vi "Measurement UI.vi"() -> ()   [LabVIEW 2021, in "audio_UI.lvlib"]
uses:
  audio_UI.lvlib
panel:
  in  "MeasGraphs":T1(tab)
  out "FreqDomainGraph":cluster{"x0":dbl, "dx":dbl, "magnitude":dbl[]}(graph) caption="AC"
  out "TimeDomainGraph":waveform(dbl)(graph) caption="AC"
  out "Channel":string
  out "Spectrum":dbl[](array[numeric])
  out "df":dbl
  out "f0":dbl
  out "Time domain":dbl[](array[numeric])
  out "dt":dbl
  out "THD+N":dbl
  out "THD":dbl
  out "SNR":dbl
  out "Calculated amplitude":dbl
  out "Calculated frequency":dbl
  out "SFDR":dbl
  out "Dynamic range":dbl
  out "Gain error":dbl
  in  "Analog source resource name":string
  in  "Protocol":string
  out "MeasTable":string[][](table)
  in  "OK Button":bool
  in  "Protocol":string(combo) caption="PROTOCOL"
  out "Calculated sample rate":u32 caption="SAMPLE RATE" format="%#.6pHz"
  in  "Protocol capture resource name":string caption="RESOURCE NAME"
  in  "Protocol settings":string="Protocol settings"
  in  "Analog source":string="Analog source "
  in  "Full scale range":dbl=3.16 caption="FULL SCALE RANGE" format="%.3pV"
  in  "Measurement settings":string="Measurement settings"
  in  "MeasSettingsOptions":i32(listbox)=-1
  in  "MeasSettings":bool
  in  "DSGResourceName":tag caption="RESOURCE NAME"
  in  "Weighting filter":T2(ring) caption="WEIGHTING FILTER"
  in  "Number of words":i32=19200 caption="NUMBER OF WORDS"
  in  "Clock rate":u32=12288000 caption="CLOCK RATE" format="%#.6pHz"
  in  "Band stop":dbl=20000.0 caption="BAND STOP" format="%#_6pHz"
  in  "Band start":dbl=20.0 caption="BAND START" format="%#_6pHz"
  in  "Amplitude":dbl=-1.0 caption="AMPLITUDE" format="%#_6pdB"
  in  "Frequency":dbl=1000.0 caption="FREQUENCY" format="%#_6pHz"
  in  "Sensitivity":dbl=0.34762 caption="SENSITIVITY" format="%.5fFS/Pa"
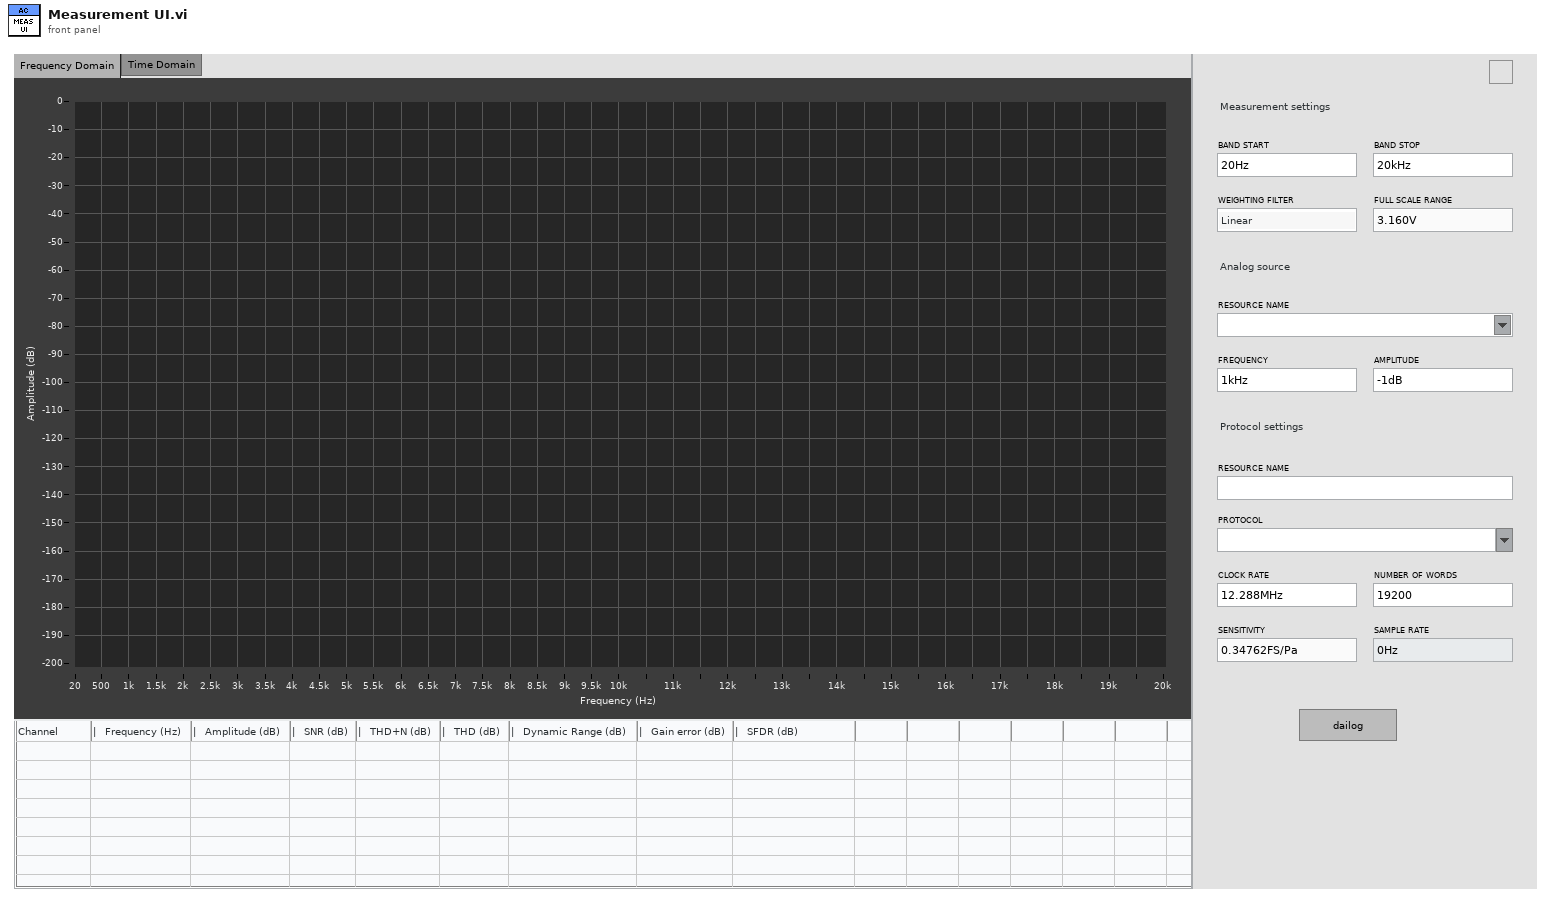
[diagram p1: front panel]
types:
  T1 = enum32{"Frequency Domain", "Time Domain", "Hidden Controls"}
  T2 = enum16{"Linear", "A-Weighting", "B-Weighting", "C-Weighting"}
  T3 = enum16{"open", "replace", "create", "open or create", "replace or create", "replace or create with confirmation"}
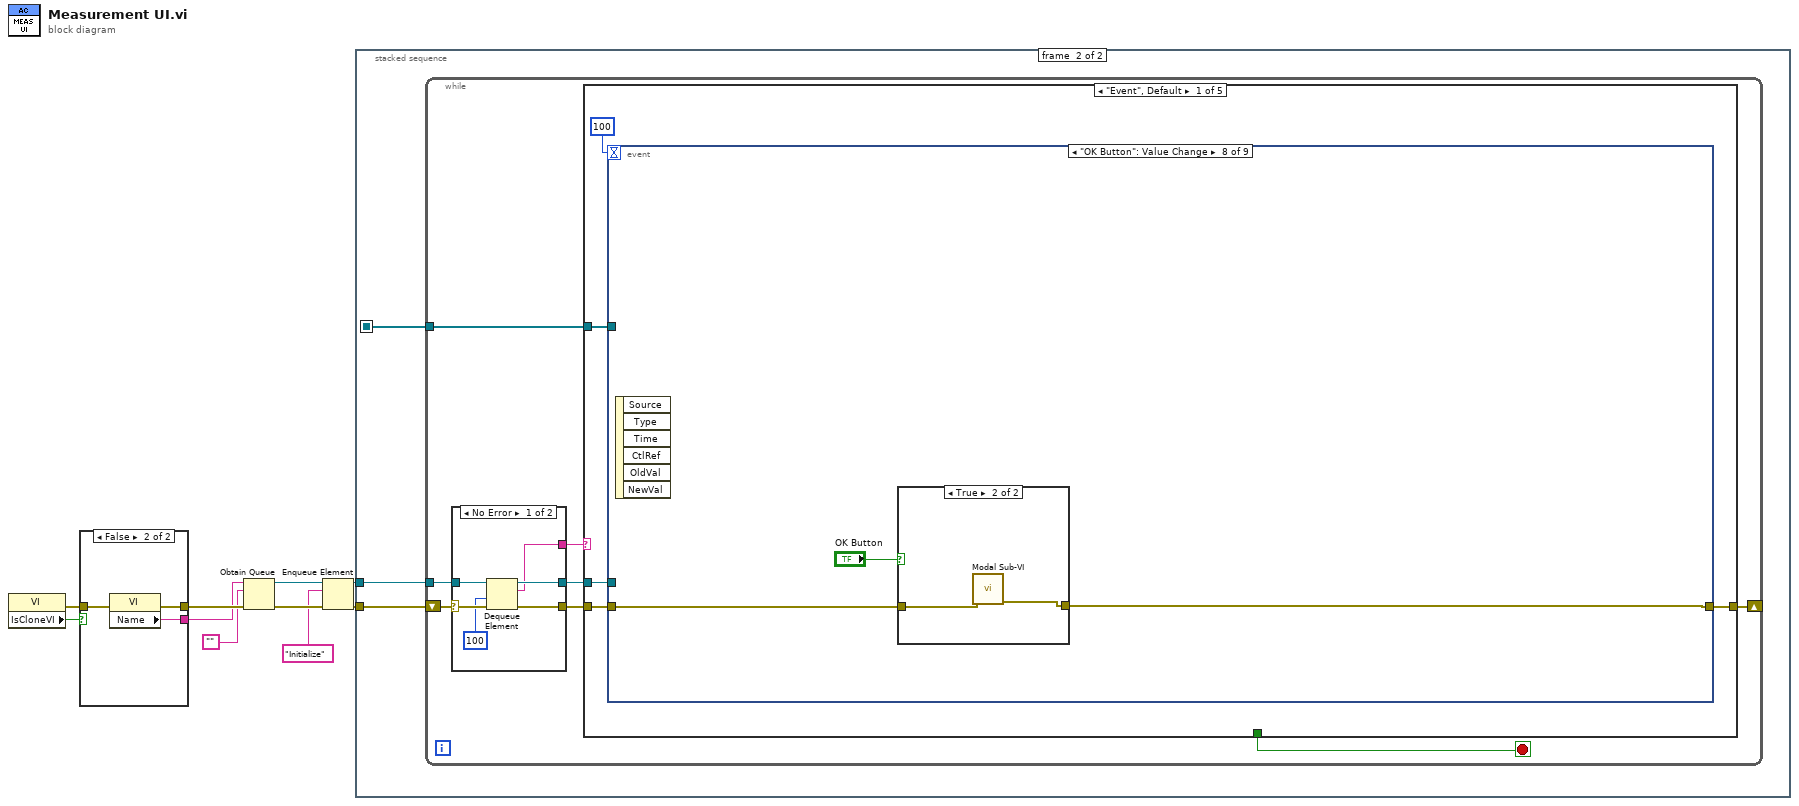
[diagram p0: block diagram]
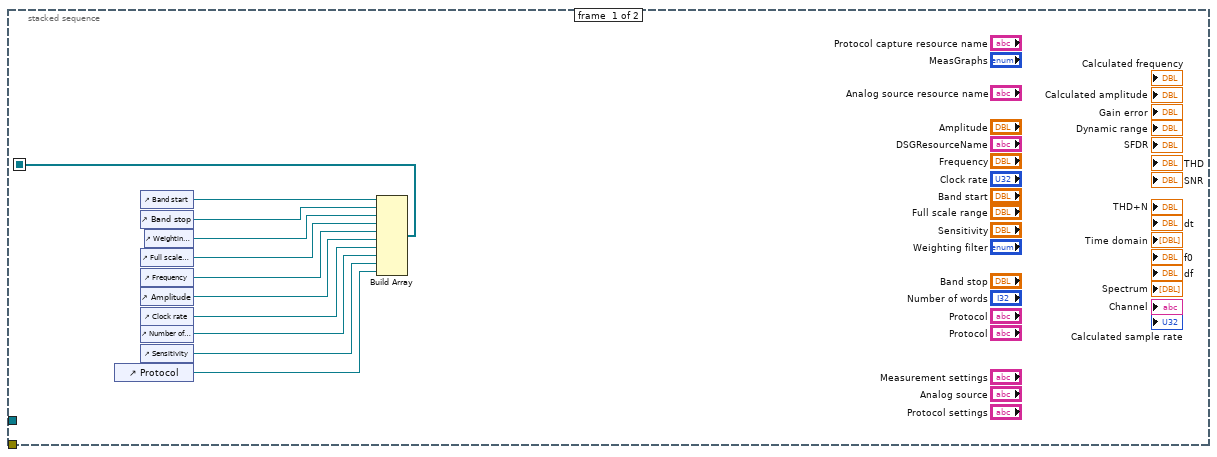
[diagram p2: hidden frame]
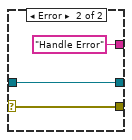
[diagram p3: hidden frame]
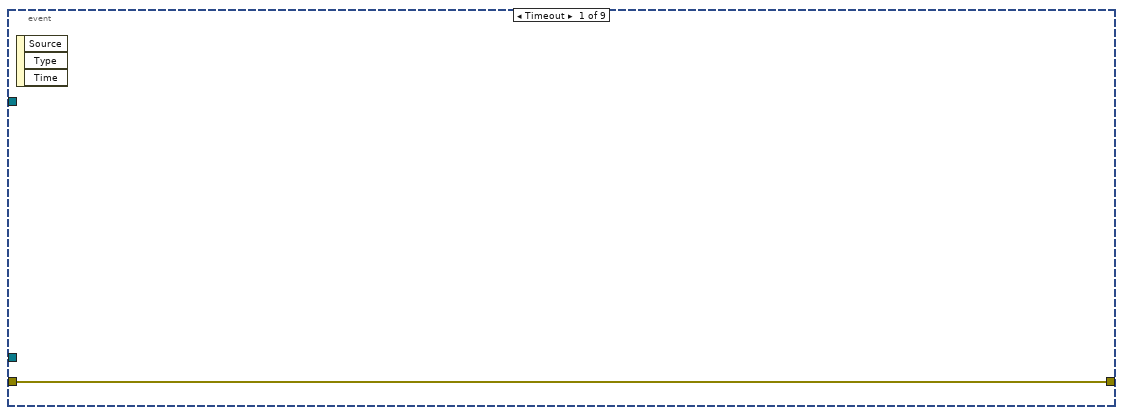
[diagram p4: hidden frame]
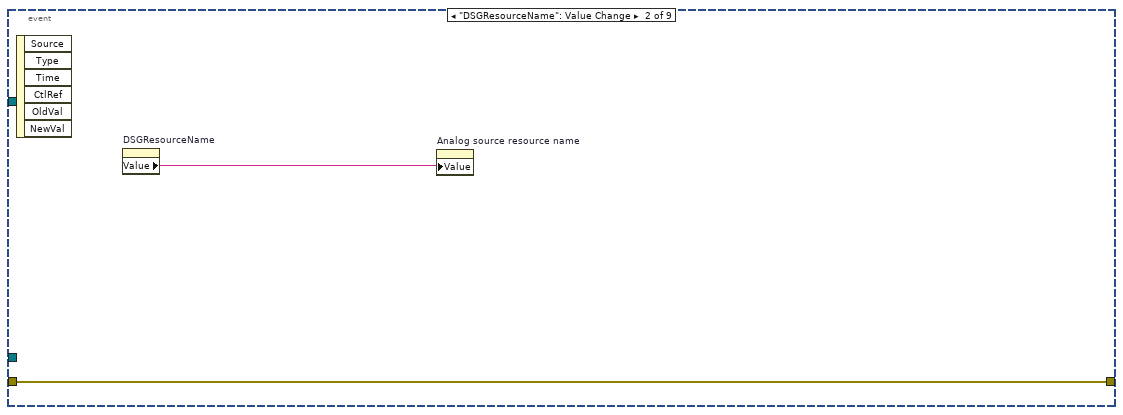
[diagram p5: hidden frame]
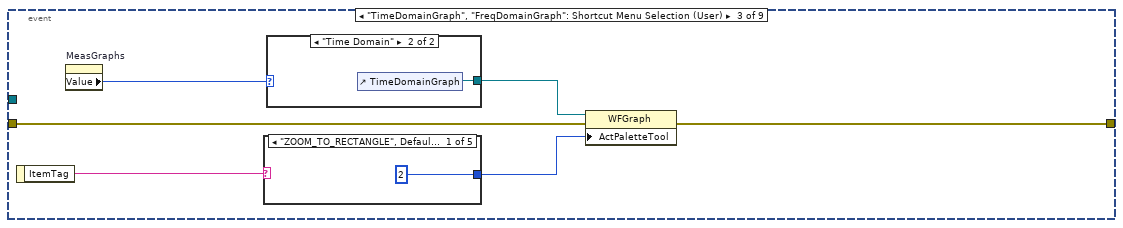
[diagram p6: hidden frame]
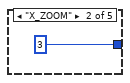
[diagram p7: hidden frame]
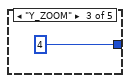
[diagram p8: hidden frame]
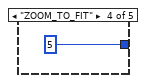
[diagram p9: hidden frame]
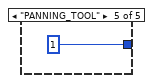
[diagram p10: hidden frame]
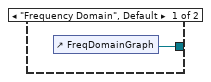
[diagram p11: hidden frame]
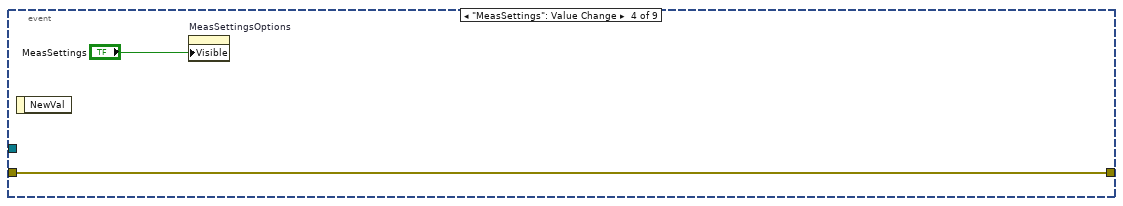
[diagram p12: hidden frame]
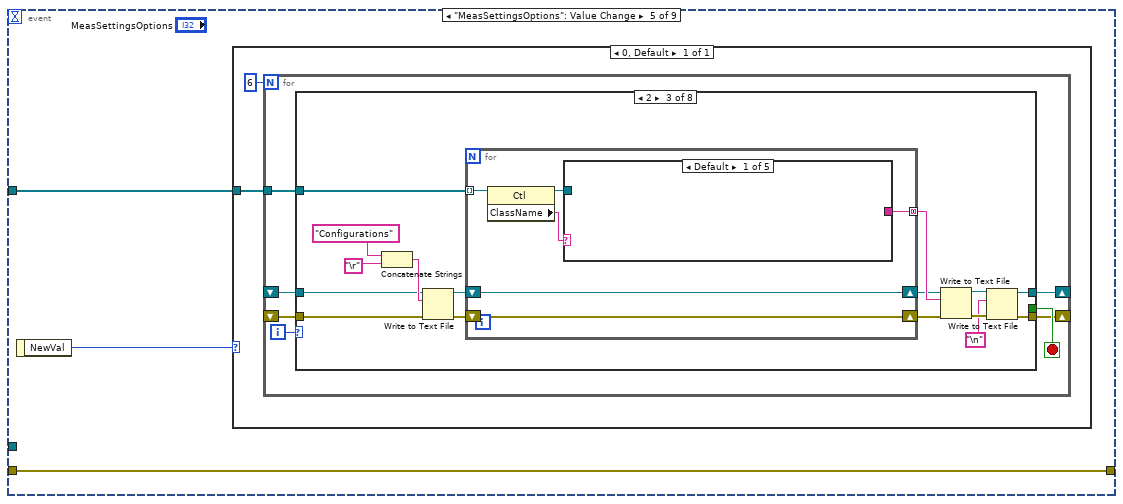
[diagram p13: hidden frame]
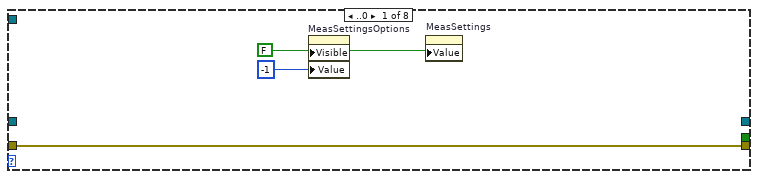
[diagram p14: hidden frame]
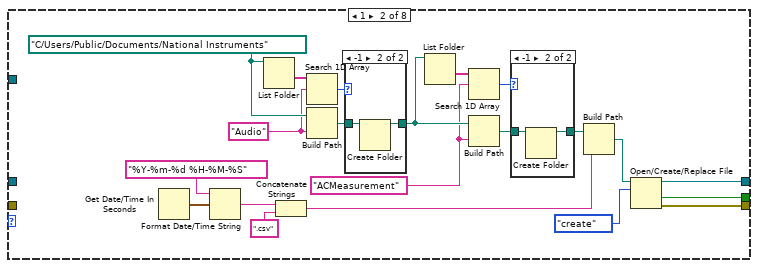
[diagram p15: hidden frame]
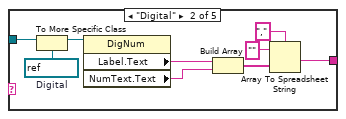
[diagram p18: hidden frame]
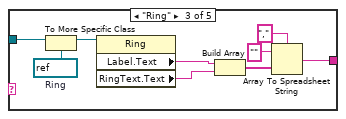
[diagram p19: hidden frame]
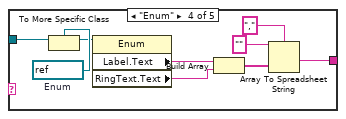
[diagram p20: hidden frame]
diagram:
  n1 = property on="Property Node" class="VI"() -> (error out=w1:errorcluster, "IsCloneVI"=w2:bool)  [unwired: 2 in, 1 out]
  n2 = case shown="False" w2 {
    tunnel: [w13 w16] -> w10
    tunnel: [w12 w15] -> w9
    tunnel: w1 -> [w11 w14]
    frame True {
      n3 = property on="Property Node" class="VI"(error in=w11) -> (error out=w13:errorcluster, "Clone Name"=w12:string)  [unwired: 1 in, 1 out]
    }
    frame False {
      n4 = property on="Property Node" class="VI"(error in=w14) -> (error out=w16:errorcluster, "Name"=w15:string)  [unwired: 1 in, 1 out]
    }
  }
  n5 = Obtain Queue(name (unnamed)=w9, element data type="" ("Empty String Constant"), error in (no error)=w10) -> (queue out=w6:refnum<queue>, error out=w8:errorcluster)  [unwired: 2 in, 1 out]
  n6 = Enqueue Element(queue=w6, element="Initialize", error in (no error)=w8) -> (queue out=w5:refnum<queue>, error out=w7:errorcluster)  [unwired: 1 in, 1 out]
  n7 = stacked-sequence {
    seq-local: [w24 _] -> [_ w28]
    tunnel: w7 -> [_ w30]
    tunnel: w5 -> [_ w29]
    frame #0 {
      n8 = control-ref of="Protocol"() -> (w17:refnum<vi>)
      n9 = control-ref of="Band start"() -> (w27:refnum<vi>)
      n10 = control-ref of="Band stop"() -> (w26:refnum<vi>)
      n11 = control-ref of="Full scale range"() -> (w23:refnum<vi>)
      n12 = control-ref of="Frequency"() -> (w22:refnum<vi>)
      n13 = control-ref of="Amplitude"() -> (w21:refnum<vi>)
      n14 = control-ref of="Clock rate"() -> (w20:refnum<vi>)
      n15 = control-ref of="Number of words"() -> (w18:refnum<vi>)
      n16 = control-ref of="Sensitivity"() -> (w19:refnum<vi>)
      n17 = control-ref of="Weighting filter"() -> (w25:refnum<vi>)
      n18 = Build Array(w27, w26, w25, w23, w22, w21, w20, w18, w19, w17) -> (w24:refnum<vi>[])
    }
    frame #1 {
      n19 = while {
        shift-right: [w33] -> _
        shift-left: w30 -> [w38]
        tunnel: w29 -> [w36]
        tunnel: w28 -> [w31]
        stop <- w32 stop-if-true
        n20 = case shown="No Error" w38 {
          selector: w38 -> [w44 w47]
          tunnel: [w43 w47] -> w37
          tunnel: w36 -> [w42 w46]
          tunnel: [w41 w46] -> w35
          tunnel: [w40 "Handle Error"] -> w34
          frame No Error {
            n21 = Dequeue Element(queue=w42, timeout in ms (-1)=100, error in (no error)=w44) -> (queue out=w41:refnum<queue>, element=w40:string, error out=w43:errorcluster)  [unwired: 1 out]
          }
          frame Error {
          }
        }
        n22 = case shown="\"Event\", Default" w34 {
          tunnel: w37 -> [w51 w325 w366 w381 w382]
          tunnel: w35 -> [w49 _ _ w379 _]
          tunnel: [w52 w325 w366 w376 w382] -> w33
          tunnel: [_ _ _ TRUE _] -> w32
          tunnel: w31 -> [w48 _ _ _ _]
          frame "Event", Default {
            n23 = event shown="[7] \"OK Button\": Value Change" {
              selector: _ -> [_ _ _ _ _ _ _ _ _]
              dyn-events: _ -> [_ _ _ _ _ _ _ _ _]
              timeout: 100 -> [_ _ _ _ _ _ _ _ _]
              tunnel: [w53 w54 w58 _ w73 w275 w279 w300 w307] -> w52
              tunnel: w51 -> [w53 w54 w57 w69 w73 w275 w278 w301 w308]
              tunnel: w49 -> [_ _ _ _ _ _ _ _ w306]
              tunnel: [_ _ _ w69 _ _ _ _ _] -> _
              tunnel: w48 -> [_ _ _ _ w71 _ _ _ _]
              event Timeout {
                n24 = event-data() -> ()  [unwired: 1 in, 3 out]
              }
              event "DSGResourceName": Value Change {
                n25 = event-data() -> ()  [unwired: 1 in, 6 out]
                n26 = property on="DSGResourceName" class="DAQmxName"() -> ("Value"=w55:string)  [unwired: 2 in, 2 out]
                n27 = property on="Analog source resource name" class="Str"("Value"=w55) -> ()  [unwired: 2 in, 2 out]
              }
              event "TimeDomainGraph", "FreqDomainGraph": Shortcut Menu Selection (User) {
                n28 = event-data() -> ("ItemTag"=w60:string)  [unwired: 1 in]
                n29 = property on="MeasGraphs" class="TabCtl (strict)"() -> ("Value"=w61:T1)  [unwired: 2 in, 2 out]
                n30 = case shown="\"ZOOM_TO_RECTANGLE\", Default" w60 {
                  tunnel: [2 3 4 5 1] -> w56
                  frame "ZOOM_TO_RECTANGLE", Default {
                  }
                  frame "X_ZOOM" {
                  }
                  frame "Y_ZOOM" {
                  }
                  frame "ZOOM_TO_FIT" {
                  }
                  frame "PANNING_TOOL" {
                  }
                }
                n31 = case shown="\"Time Domain\"" w61 {
                  tunnel: [w67 w68] -> w59
                  frame "Frequency Domain", Default {
                    n32 = control-ref of="FreqDomainGraph"() -> (w67:refnum<vi>)
                  }
                  frame "Time Domain" {
                    n33 = control-ref of="TimeDomainGraph"() -> (w68:refnum<vi>)
                  }
                }
                n34 = property on="Property Node" class="WFGraph"(reference=w59, error in=w57, "ActPaletteTool"=w56) -> (error out=w58:errorcluster)  [unwired: 1 out]
              }
              event "MeasSettings": Value Change {
                n35 = event-data() -> ()  [unwired: 1 in, 1 out]
                n36 = property on="MeasSettingsOptions" class="LstBox (strict)"("Visible"="MeasSettings") -> ()  [unwired: 2 in, 2 out]
              }
              event "MeasSettingsOptions": Value Change {
                n37 = event-data() -> ("NewVal"=w72:i32)  [unwired: 1 in]
                n38 = case shown="0, Default" w72 {
                  tunnel: w71 -> [w74]
                  frame 0, Default {
                    n39 = for {
                      N: 6 -> [_]
                      shift-right: [w80] -> _
                      shift-left: _ -> [w79]
                      shift-right: [w78] -> _
                      shift-left: _ -> [w77]
                      tunnel: w74 -> [w76]
                      i -> [w82]
                      stop <- w81 stop-if-true
                      n40 = case shown="2" w82 {
                        tunnel: [_ w99 _ _ _ _ _ _] -> w81
                        tunnel: [_ w105 w125 w178 w205 w246 refnum<file> refnum ("refnum out") w274] -> w80
                        tunnel: w79 -> [_ _ w122 w189 w228 w247 w272 w274]
                        tunnel: [w83 w98 w124 w177 w203 w245 w270 w273] -> w78
                        tunnel: w77 -> [w83 _ w120 w188 w227 w248 w269 w273]
                        tunnel: w76 -> [_ _ w123 _ _ _ _ _]
                        frame ..0 {
                          w85 = FALSE ("Visible")
                          n41 = property on="MeasSettingsOptions" class="LstBox (strict)"("Visible"=w85, "Value"=-1 ("MeasSettingsOptions")) -> ()  [unwired: 2 in, 2 out]
                          n42 = property on="MeasSettings" class="Bool (strict)"("Value"=w85) -> ()  [unwired: 2 in, 2 out]
                        }
                        frame 1 {
                          w94 = "ACMeasurement" ("prompt")
                          w101 = "Audio" ("prompt")
                          w104 = path "C:/Users/Public/Documents/National Instruments" ("base path")
                          n43 = Get Date/Time In Seconds() -> (seconds since 1Jan1904=w91:timestamp)
                          n44 = Format Date/Time String(time format string (%c)="%Y-%m-%d %H-%M-%S", seconds (now)=w91) -> (date/time string=w90:string)  [unwired: 1 in]
                          n45 = List Folder(path=w104) -> (folder names=w102:string[])  [unwired: 3 in, 3 out]
                          n46 = Concatenate Strings(w90, ".csv" ("string")) -> (w87:string)
                          n47 = Search 1D Array(1D array=w102, element=w101) -> (index of element=w100:i32)  [unwired: 1 in]
                          n48 = Build Path(base path=w104, name or relative path=w101) -> (appended path=w103:path)
                          n49 = case shown="-1" w100 {
                            tunnel: w103 -> [w110 w112]
                            tunnel: [w110 w111] -> w95
                            frame Default {
                            }
                            frame -1 {
                              n50 = Create Folder(path (use dialog)=w112) -> (created path=w111:path)  [unwired: 2 in, 2 out]
                            }
                          }
                          n51 = List Folder(path=w95) -> (folder names=w97:string[])  [unwired: 3 in, 3 out]
                          n52 = Search 1D Array(1D array=w97, element=w94) -> (index of element=w96:i32)  [unwired: 1 in]
                          n53 = Build Path(base path=w95, name or relative path=w94) -> (appended path=w93:path)
                          n54 = case shown="-1" w96 {
                            tunnel: w93 -> [w107 w109]
                            tunnel: [w107 w108] -> w88
                            frame Default {
                            }
                            frame -1 {
                              n55 = Create Folder(path (use dialog)=w109) -> (created path=w108:path)  [unwired: 2 in, 2 out]
                            }
                          }
                          n56 = Build Path(base path=w88, name or relative path=w87) -> (appended path=w86:path)
                          n57 = Open/Create/Replace File(file path (use dialog)=w86, operation (0:open)=T3."create") -> (refnum out=w105:refnum<file>, cancelled=w99:bool, error out=w98:errorcluster)  [unwired: 4 in]
                        }
                        frame 2 {
                          n58 = Concatenate Strings("Configurations" ("format string"), "\r" ("Carriage Return Constant")) -> (w126:string)
                          n59 = Write to Text File(file (use dialog)=w122, text=w126, error in=w120) -> (refnum out=w119:refnum<file>, error out=w121:errorcluster)  [unwired: 1 in, 1 out]
                          n60 = for {
                            tunnel: w123 -> [w130] mode=indexing
                            shift-right: [w134] -> w117
                            shift-left: w119 -> [w134]
                            shift-right: [w133] -> w116
                            shift-left: w121 -> [w133]
                            tunnel: [w132] -> w118 mode=concatenating
                            n61 = property on="Property Node" class="Ctl"(reference=w130) -> (reference out=w131:refnum<vi>, "ClassName"=w129:string)  [unwired: 1 in, 1 out]
                            n62 = case shown="Default" w129 {
                              tunnel: [_ w138 w148 w157 w162] -> w132
                              tunnel: w131 -> [_ w136 w146 w161 w170]
                              frame Default {
                              }
                              frame "Digital" {
                                w135 = refnum<vi> refnum  # Digital
                                n63 = To More Specific Class(target class=w135, reference=w136) -> (specific class reference=w137:refnum<vi>)  [unwired: 1 in, 1 out]
                                n64 = property on="Property Node" class="DigNum"(reference=w137) -> ("Label.Text"=w143:string, "NumText.Text"=w142:string)  [unwired: 1 in, 2 out]
                                n65 = Build Array(w143, w142) -> (w139:string[])
                                n66 = Array To Spreadsheet String(delimiter (Tab)=",", array=w139, 3:"" ("format string")) -> (spreadsheet string=w138:string)
                              }
                              frame "Ring" {
                                w145 = refnum<vi> refnum  # Ring
                                n67 = To More Specific Class(target class=w145, reference=w146) -> (specific class reference=w147:refnum<vi>)  [unwired: 1 in, 1 out]
                                n68 = property on="Property Node" class="Ring"(reference=w147) -> ("Label.Text"=w144:string, "RingText.Text"=w152:string)  [unwired: 1 in, 2 out]
                                n69 = Build Array(w144, w152) -> (w149:string[])
                                n70 = Array To Spreadsheet String(delimiter (Tab)=",", array=w149, 3:"" ("format string")) -> (spreadsheet string=w148:string)
                              }
                              frame "Enum" {
                                w160 = refnum<vi> refnum  # Enum
                                n71 = To More Specific Class(target class=w160, reference=w161) -> (specific class reference=w156:refnum<vi>)  [unwired: 1 in, 1 out]
                                n72 = property on="Property Node" class="Enum"(reference=w156) -> ("Label.Text"=w155:string, "RingText.Text"=w154:string)  [unwired: 1 in, 2 out]
                                n73 = Build Array(w155, w154) -> (w153:string[])
                                n74 = Array To Spreadsheet String(delimiter (Tab)=",", array=w153, 3:"" ("format string")) -> (spreadsheet string=w157:string)
                              }
                              frame "ComboBox" {
                                w169 = refnum<vi> refnum  # ComboBox
                                n75 = To More Specific Class(target class=w169, reference=w170) -> (specific class reference=w168:refnum<vi>)  [unwired: 1 in, 1 out]
                                n76 = property class="CmbBox"(reference=w168) -> ("Label.Text"=w164:string, "Value"=w163:string)  [unwired: 1 in, 2 out]
                                n77 = Build Array(w164, w163) -> (w167:string[])
                                n78 = Array To Spreadsheet String(delimiter (Tab)=",", array=w167, 3:"" ("format string")) -> (spreadsheet string=w162:string)
                              }
                            }
                          }
                          n79 = Write to Text File(file (use dialog)=w117, text=w118, error in=w116) -> (refnum out=w115:refnum<file>, error out=w114:errorcluster)  [unwired: 1 in, 1 out]
                          n80 = Write to Text File(file (use dialog)=w115, text="\n" ("Line Feed Constant"), error in=w114) -> (refnum out=w125:refnum<file>, error out=w124:errorcluster)  [unwired: 1 in, 1 out]
                        }
                        frame 3 {
                          n81 = property on="MeasTable" class="Tbl (strict)"() -> ("Column Headers[]"=w172:string[], "Value"=w171:string[][])  [unwired: 2 in, 2 out]
                          n82 = Build Array (concatenate)(w172, w171) -> (w186:string[][])
                          n83 = for {
                            tunnel: w186 -> [w191] mode=indexing
                            tunnel: [w190] -> w185 mode=indexing
                            n84 = for {
                              tunnel: w191 -> [w193] mode=indexing
                              tunnel: [w192] -> w190 mode=indexing
                              n85 = Match Pattern(string=w193, regular expression="|") -> (before substring=w197:string, after substring=w196:string, offset past match=w199:i32)  [unwired: 1 in, 1 out]
                              n86 = Less Than 0?(x=w199) -> (x < 0?=w198:bool)
                              n87 = Select(t=w197, s=w198, f=w196) -> (s? t:f=w195:string)
                              n88 = Match Pattern(string=w195, regular expression="[\\t\\n\\r\\s]*$") -> (before substring=w192:string)  [unwired: 1 in, 3 out]
                            }
                          }
                          n89 = Concatenate Strings("Results" ("element"), "\r" ("Carriage Return Constant")) -> (w173:string)
                          n90 = Write to Text File(file (use dialog)=w189, text=w173, error in=w188) -> (refnum out=w187:refnum<file>, error out=w181:errorcluster)  [unwired: 1 in, 1 out]
                          n91 = Array To Spreadsheet String(delimiter (Tab)=",", array=w185, 3:"" ("format string")) -> (spreadsheet string=w182:string)
                          n92 = Write to Text File(file (use dialog)=w187, text=w182, error in=w181) -> (refnum out=w180:refnum<file>, error out=w179:errorcluster)  [unwired: 1 in, 1 out]
                          n93 = Write to Text File(file (use dialog)=w180, text="\n" ("Line Feed Constant"), error in=w179) -> (refnum out=w178:refnum<file>, error out=w177:errorcluster)  [unwired: 1 in, 1 out]
                        }
                        frame 4 {
                          n94 = property on="FreqDomainGraph" class="WFGraph (strict)"() -> ("Value"=w208:cluster{"x0":dbl, "dx":dbl, "magnitude":dbl[]})  [unwired: 2 in, 2 out]
                          n95 = Concatenate Strings("Frequency Domain" ("string"), "\r" ("Carriage Return Constant")) -> (w225:string)
                          n96 = Build Array("Frequency (Hz)", "Amplitude (dB)") -> (w224:string[])
                          n97 = Write to Text File(file (use dialog)=w228, text=w225, error in=w227) -> (refnum out=w221:refnum<file>, error out=w220:errorcluster)  [unwired: 1 in, 1 out]
                          n98 = Unbundle By Name(w208) -> ("dx"=w212:dbl, "x0"=w213:dbl, "magnitude"=w211:dbl[])
                          n99 = Array To Spreadsheet String(delimiter (Tab)=",", array=w224, 3:"" ("format string")) -> (spreadsheet string=w219:string)
                          n100 = Write to Text File(file (use dialog)=w221, text=w219, error in=w220) -> (refnum out=w218:refnum<file>, error out=w217:errorcluster)  [unwired: 1 in, 1 out]
                          n101 = for {
                            tunnel: w211 -> [w232] mode=indexing
                            tunnel: w212 -> [w236]
                            tunnel: w213 -> [w234]
                            tunnel: [w229] -> w214 mode=indexing
                            i -> [w237]
                            n102 = Multiply(x=w237, y=w236) -> (x*y=w235:dbl)
                            n103 = Add(x=w235, y=w234) -> (x+y=w233:dbl)
                            n104 = Format Into String(w233) -> (resulting string=w230:string)  [unwired: 3 in, 1 out]
                            n105 = Format Into String(w232) -> (resulting string=w231:string)  [unwired: 3 in, 1 out]
                            n106 = Build Array(w230, w231) -> (w229:string[])
                          }
                          n107 = Array To Spreadsheet String(delimiter (Tab)=",", array=w214, 3:"" ("format string")) -> (spreadsheet string=w210:string)
                          n108 = Write to Text File(file (use dialog)=w218, text=w210, error in=w217) -> (refnum out=w207:refnum<file>, error out=w206:errorcluster)  [unwired: 1 in, 1 out]
                          n109 = Write to Text File(file (use dialog)=w207, text="\n" ("Line Feed Constant"), error in=w206) -> (refnum out=w205:refnum<file>, error out=w203:errorcluster)  [unwired: 1 in, 1 out]
                        }
                        frame 5 {
                          n110 = property on="TimeDomainGraph" class="WFGraph (strict)"() -> ("Value"=w244:waveform(dbl))  [unwired: 2 in, 2 out]
                          n111 = Concatenate Strings("Time Domain" ("string"), "\r" ("Carriage Return Constant")) -> (w260:string)
                          n112 = Write to Text File(file (use dialog)=w247, text=w260, error in=w248) -> (refnum out=w257:refnum<file>, error out=w256:errorcluster)  [unwired: 1 in, 1 out]
                          n113 = Build Array("Time (s)", "Amplitude (V)") -> (w259:string[])
                          n114 = Unbundle By Name ("Get Waveform Components")(w244) -> ("dt"=w242:dbl, "Y"=w243:dbl[])
                          n115 = Array To Spreadsheet String(delimiter (Tab)=",", array=w259, 3:"" ("format string")) -> (spreadsheet string=w255:string)
                          n116 = Write to Text File(file (use dialog)=w257, text=w255, error in=w256) -> (refnum out=w254:refnum<file>, error out=w253:errorcluster)  [unwired: 1 in, 1 out]
                          n117 = for {
                            tunnel: [w266] -> w250 mode=indexing
                            tunnel: w243 -> [w265] mode=indexing
                            tunnel: w242 -> [w263]
                            i -> [w264]
                            n118 = Multiply(x=w263, y=w264) -> (x*y=w262:dbl)
                            n119 = Format Into String(w262) -> (resulting string=w267:string)  [unwired: 3 in, 1 out]
                            n120 = Format Into String(w265) -> (resulting string=w268:string)  [unwired: 3 in, 1 out]
                            n121 = Build Array(w267, w268) -> (w266:string[])
                          }
                          n122 = Array To Spreadsheet String(delimiter (Tab)=",", array=w250, 3:"" ("format string")) -> (spreadsheet string=w249:string)
                          n123 = Write to Text File(file (use dialog)=w254, text=w249, error in=w253) -> (refnum out=w246:refnum<file>, error out=w245:errorcluster)  [unwired: 1 in, 1 out]
                        }
                        frame 6 {
                          n124 = Close File(refnum=w272, error in=w269) -> (error out=w270:errorcluster)  [unwired: 1 out]
                        }
                        frame Default {
                        }
                      }
                    }
                  }
                }
              }
              event Mouse Down {
                w276 = FALSE ("Visible")
                n125 = event-data() -> ()  [unwired: 1 in, 1 out]
                n126 = property on="MeasSettingsOptions" class="LstBox (strict)"("Visible"=w276, "Value"=-1 ("MeasSettingsOptions")) -> ()  [unwired: 2 in, 2 out]
                n127 = property on="MeasSettings" class="Bool (strict)"("Value"=w276) -> ()  [unwired: 2 in, 2 out]
              }
              event "Protocol": Value Change {
                n128 = event-data() -> ()  [unwired: 1 in, 1 out]
                n129 = property on="Protocol" class="CmbBox"() -> ("Value"=w280:string)  [unwired: 2 in, 2 out]
                n130 = case shown="\"Refresh\"" w280 {
                  tunnel: w280 -> [w282 _]
                  tunnel: [w281 w285] -> w279
                  tunnel: w278 -> [w281 w284]
                  frame Default {
                    n131 = property on="Protocol" class="Str"("Value"=w282) -> ()  [unwired: 2 in, 2 out]
                  }
                  frame "Refresh" {
                    n132 = List Folder(path=path "C:/Users/Public/Documents/National Instruments/Audio/Protocols", error in=w284) -> (filenames=w295:string[])  [unwired: 2 in, 3 out]
                    n133 = for {
                      tunnel: w295 -> [w297] mode=indexing
                      tunnel: [w296] -> w293 mode=indexing
                      n134 = Search/Split String(string=w297, search string/char (-)=".JSON") -> (substring before match=w296:string)  [unwired: 1 in, 2 out]
                    }
                    n135 = Insert Into Array(array=w293, index=0, new element="Refresh" ("new element/subarray")) -> (w290:string[])
                    n136 = Insert Into Array(array=w290, index=1, new element="-" ("new element/subarray")) -> (w287:string[])
                    n137 = property on="Protocol" class="CmbBox"("Strings[]"=w287) -> (error out=w286:errorcluster)  [unwired: 2 in, 1 out]
                    n138 = property on="Protocol" class="CmbBox"(error in=w286, "Value"="" ("Protocol")) -> (error out=w285:errorcluster)  [unwired: 1 in, 1 out]
                  }
                }
              }
              event "OK Button": Value Change {
                n139 = event-data() -> ()  [unwired: 1 in, 6 out]
                n140 = case shown="True" "OK Button" {
                  tunnel: w301 -> [w302 w304]
                  tunnel: [w302 w303] -> w300
                  frame False {
                  }
                  frame True {
                    n141 = call "Modal Sub-VI.vi"("error in (no error)"=w304) -> ("error out"=w303:errorcluster)  [unwired: 10 in]
                  }
                }
              }
              event Panel Close? {
                n142 = event-data() -> ()  [unwired: 1 in, 4 out]
                n143 = Enqueue Element(queue=w306, element="Exit", error in (no error)=w308) -> (error out=w307:errorcluster)  [unwired: 1 in, 2 out]
                n144 = event-data ("Event Filter Node")("Discard?"=TRUE) -> ()  [unwired: 1 in, 1 out]
              }
            }
          }
          frame "Initialize" {
            w323 = string[] ["Export data"] ("Item Names")
            n145 = for {
              N: 2 -> [_]
              i -> [w331]
              n146 = case shown="1" w331 {
                tunnel: [w334 w335] -> w332
                frame 0, Default {
                  n147 = control-ref of="FreqDomainGraph"() -> (w334:refnum<vi>)
                }
                frame 1 {
                  n148 = control-ref of="TimeDomainGraph"() -> (w335:refnum<vi>)
                }
              }
              n149 = property on="Property Node" class="WFGraph"(reference=w332, "ActPaletteTool"=2 ("Palette:Active Tool")) -> ()  [unwired: 1 in, 2 out]
            }
            n150 = property on="DSGResourceName" class="DAQmxName"("Value"="<Select Device>") -> ()  [unwired: 2 in, 2 out]
            n151 = List Folder(path=path "C:/Users/Public/Documents/National Instruments/Audio/Protocols") -> (filenames=w318:string[])  [unwired: 3 in, 3 out]
            n152 = for {
              tunnel: w318 -> [w327] mode=indexing
              tunnel: [w326] -> w316 mode=indexing
              n153 = Search/Split String(string=w327, search string/char (-)=".JSON") -> (substring before match=w326:string)  [unwired: 1 in, 2 out]
            }
            n154 = property on="MeasSettingsOptions" class="LstBox (strict)"("Item Names"=w323, "Value"=-1 ("MeasSettingsOptions"), "Visible"=FALSE, "Disabled Items"=i32[] []) -> ()  [unwired: 2 in, 2 out]
            n155 = Insert Into Array(array=w316, index=0, new element="Refresh" ("new element/subarray")) -> (w313:string[])
            n156 = for {
              tunnel: w323 -> [_] mode=indexing
              i -> [w330]
              n157 = property on="MeasSettingsOptions" class="LstBox (strict)"("Active Row"=w330, "Cell Height"=30 ("Active Row:Cell Height")) -> ()  [unwired: 2 in, 2 out]
            }
            n158 = Insert Into Array(array=w313, index=1, new element="-" ("new element/subarray")) -> (w310:string[])
            n159 = property on="Protocol" class="CmbBox"("Strings[]"=w310) -> ()  [unwired: 2 in, 2 out]
          }
          frame "Post UI Update" {
            w348 = "|   " ("initial string")
            # "This case will be triggered, after framework updates the User interface with result values."
            n160 = local read "Time domain"() -> (w365:dbl[])
            n161 = local read "Spectrum"() -> (w339:dbl[])
            n162 = local read "df"() -> (w341:dbl)
            n163 = local read "dt"() -> (w364:dbl)
            n164 = local read "f0"() -> (w338:dbl)
            n165 = local read "Calculated frequency"() -> (w351:dbl)
            n166 = local read "Calculated amplitude"() -> (w350:dbl)
            n167 = local read "Dynamic range"() -> (w360:dbl)
            n168 = Bundle By Name ("Build Waveform")("Y"=w365, "dt"=w364) -> (→"TimeDomainGraph":waveform(dbl))  [unwired: 1 in]
            n169 = Bundle(cluster=cluster{"x0":dbl, "dx":dbl, "magnitude":dbl[]} {"x0"=0.0, "dx"=0.0, "magnitude"=[]} ("FreqDomainGraph"), "x0"=w338, "dx"=w341, "magnitude"=w339) -> (→"FreqDomainGraph":cluster{"x0":dbl, "dx":dbl, "magnitude":dbl[]})
            n170 = local read "THD+N"() -> (w361:dbl)
            n171 = local read "Gain error"() -> (w347:dbl)
            n172 = local read "THD"() -> (w362:dbl)
            n173 = local read "SNR"() -> (w349:dbl)
            n174 = local read "SFDR"() -> (w346:dbl)
            n175 = Build Array(w351, w350) -> (w357:dbl[])
            n176 = Build Array(w349, w361, w362, w360) -> (w356:dbl[])
            n177 = for {
              tunnel: w357 -> [w371] mode=indexing
              tunnel: w348 -> [w372]
              tunnel: "%.3f" ("initial string") -> [w373]
              tunnel: [w374] -> w355 mode=indexing
              n178 = Format Into String(format string=w373, initial string=w372, w371) -> (resulting string=w374:string)  [unwired: 1 in, 1 out]
            }
            n179 = for {
              tunnel: w356 -> [w367] mode=indexing
              tunnel: w348 -> [w368]
              tunnel: "%5.1f" ("initial string") -> [w369]
              tunnel: [w370] -> w354 mode=indexing
              n180 = Format Into String(format string=w369, initial string=w368, w367) -> (resulting string=w370:string)  [unwired: 1 in, 1 out]
            }
            n181 = Format Into String(format string="%5.1f" ("initial string"), initial string=w348, w346) -> (resulting string=w344:string)  [unwired: 1 in, 1 out]
            n182 = Format Into String(format string="%5.3f" ("initial string"), initial string=w348, w347) -> (resulting string=w345:string)  [unwired: 1 in, 1 out]
            n183 = local read "Channel"() -> (w336:string)
            n184 = Build Array (concatenate)(w336, w355, w354, w345, w344) -> (w353:string[])
            n185 = Build Array(w353) -> (→"MeasTable":string[][])
          }
          frame "Exit" {
            # "This case is triggered to close the User Interface from framework"
            n186 = Flush Queue(queue=w379, error in (no error)=w381) -> (queue out=w378:refnum<queue>, error out=w377:errorcluster)  [unwired: 1 out]
            n187 = Release Queue(queue=w378, force destroy? (F)=TRUE, error in (no error)=w377) -> (error out=w376:errorcluster)  [unwired: 2 out]
          }
          frame "Handle Error" {
          }
        }
      }
    }
  }
